vi "Foward Kinematics.vi"(10 "Encoder Position":dbl[](array[numeric]), 11 "Motor Configuration":dbl[][](array[numeric])) -> (3 "Measured Position":dbl[](array[numeric]))   [LabVIEW 2021]
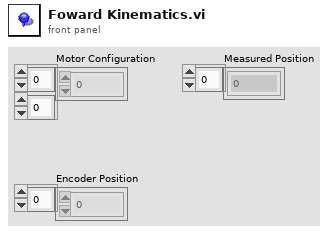
[diagram p1: front panel]
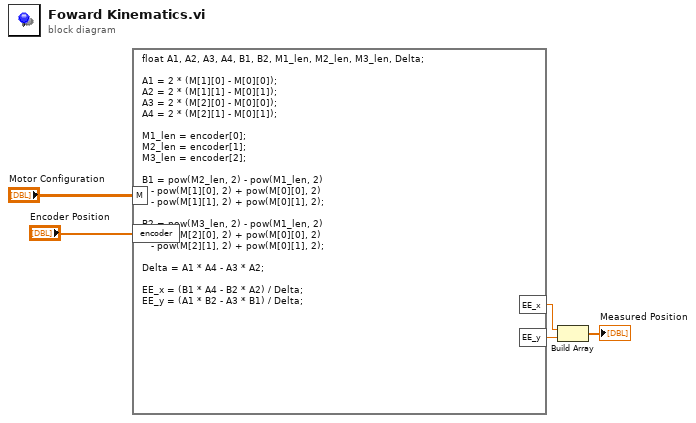
[diagram p0: block diagram]
diagram:
  n1 = formula code="float A1, A2, A3, A4, B1, B2, M1_len, M2_len, M3_len, Delta;\n\nA1 = 2 * (M[1][0] - M[0][0]);\nA2 = 2 * (M[1][1] - M[0][1]);\nA3 = 2 * (M[2][0] - M[0][0]);\nA4 = 2 * (M[2][1] - M[0][1]);\n\nM1_len = encoder[0]; \nM2_len = encoder[1];\nM3_len = encoder[2];\n\nB1 = pow(M2_len, 2) - pow(M1_len, 2)\n   - pow(M[1][0], 2) + pow(M[0][0], 2)\n   - pow(M[1][1], 2) + pow(M[0][1], 2);\n\nB2 = pow(M3_len, 2) - pow(M1_len, 2)\n   - pow(M[2][0], 2) + pow(M[0][0], 2)\n   - pow(M[2][1], 2) + pow(M[0][1], 2);\n\nDelta = A1 * A4 - A3 * A2;\n\nEE_x = (B1 * A4 - B2 * A2) / Delta;\nEE_y = (A1 * B2 - A3 * B1) / Delta;"("M"="Motor Configuration", "encoder"="Encoder Position") -> ("EE_x"=w3:dbl, "EE_y"=w4:dbl)
  n2 = Build Array(w3, w4) -> (→"Measured Position":dbl[])
